vi "4461 timing test.vi"() -> ()   [LabVIEW 2015]
uses:
  <vilib>/DAQmx/write.llb/DAQmx Write (Analog 1D DBL 1Chan NSamp).vi
  <vilib>/DAQmx/create/channels.llb/DAQmx Create Channel (AO-Voltage-Basic).vi
  <vilib>/DAQmx/configure/timing.llb/DAQmx Timing (Sample Clock).vi
  <vilib>/DAQmx/configure/trigger.llb/DAQmx Start Trigger (Digital Edge).vi
  <vilib>/DAQmx/miscellaneous.llb/DAQmx Fill In Error Info.vi
  <resource>/objmgr/daqmx.rc
  <vilib>/Analysis/NI_AALBase.lvlib
panel:
  in  "stop":bool
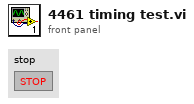
[diagram p1: front panel]
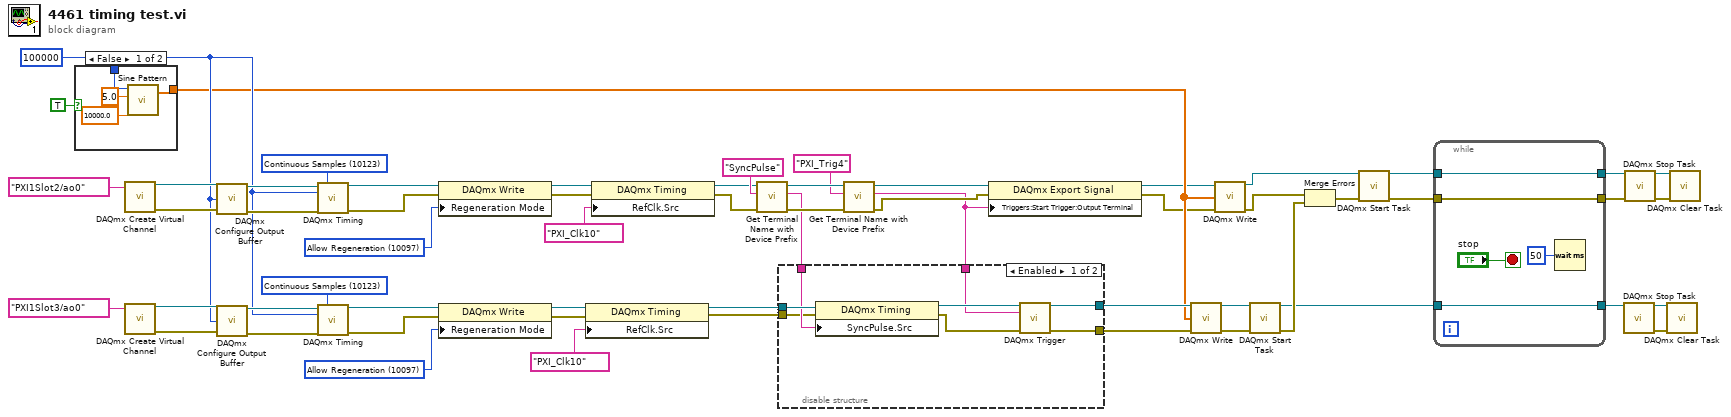
[diagram p0: block diagram]
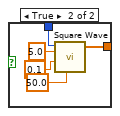
[diagram p2: hidden frame]
diagram:
  w31 = 10123 items=["Finite Samples"=10178, "Continuous Samples"=10123, "Hardware Timed Single Point"=12522] ("sample mode")
  w35 = 10097 items=["Allow Regeneration"=10097, "Do Not Allow Regeneration"=10158] ("RegenMode")
  w30 = 100000
  w51 = 10123 items=["Finite Samples"=10178, "Continuous Samples"=10123, "Hardware Timed Single Point"=12522] ("sample mode")
  w55 = 10097 items=["Allow Regeneration"=10097, "Do Not Allow Regeneration"=10158] ("RegenMode")
  n1 = case shown="False" TRUE {
    tunnel: w30 -> [w62 w68]
    tunnel: [w63 w67] -> w6
    frame False {
      n2 = call <vilib>:"Sine Pattern.vi"("cycles"=10000.0, "amplitude"=5.0, "samples"=w62) -> ("Sinusoidal Pattern"=w63:dbl[])  [unwired: 1 in, 1 out]
    }
    frame True {
      n3 = call <vilib>:"Square Wave.vi"("samples"=w68, "amplitude"=5.0, "frequency"=0.1 ("cycles"), "duty cycle (%)"=50.0) -> ("square wave"=w67:dbl[])  [unwired: 2 in, 2 out]
    }
  }
  n4 = call-poly <vilib>:"DAQmx Create Virtual Channel.vi"("physical channels"=tag "PXI1Slot2/ao0") -> ("task out"=w59:refnum<k21>, "error out"=w54:errorcluster)  [unwired: 13 in]
  n5 = call-poly <vilib>:"DAQmx Create Virtual Channel.vi"("physical channels"=tag "PXI1Slot3/ao0") -> ("task out"=w39:refnum<k21>, "error out"=w34:errorcluster)  [unwired: 13 in]
  n6 = call <vilib>:"DAQmx Configure Output Buffer.vi"("task/channels in"=w59, "buffer size (in samples per channel)"=w30, "error in"=w54) -> ("task out"=w58:refnum<k21>, "error out"=w53:errorcluster)  [unwired: 11 in]
  n7 = call <vilib>:"DAQmx Configure Output Buffer.vi"("task/channels in"=w39, "buffer size (in samples per channel)"=w30, "error in"=w34) -> ("task out"=w38:refnum<k21>, "error out"=w33:errorcluster)  [unwired: 11 in]
  n8 = call-poly <vilib>:"DAQmx Timing.vi"("task/channels in"=w58, "sample mode"=w51, "rate"=w30, "error in"=w53) -> ("task out"=w56:refnum<k21>, "error out"=w57:errorcluster)  [unwired: 10 in]
  n9 = call-poly <vilib>:"DAQmx Timing.vi"("task/channels in"=w38, "sample mode"=w31, "rate"=w30, "error in"=w33) -> ("task out"=w36:refnum<k21>, "error out"=w37:errorcluster)  [unwired: 10 in]
  n10 = property class="DAQmx Write"(reference=w56, error in=w57, "Regeneration Mode"=w55) -> (reference out=w41:refnum<k21>, error out=w40:errorcluster)
  n11 = property class="DAQmx Write"(reference=w36, error in=w37, "Regeneration Mode"=w35) -> (reference out=w28:refnum<k21>, error out=w27:errorcluster)
  n12 = property class="DAQmx Timing"(reference=w28, error in=w27, "RefClk.Src"=tag "PXI_Clk10") -> (reference out=w26:refnum<k21>, error out=w24:errorcluster)
  n13 = property class="DAQmx Timing"(reference=w41, error in=w40, "RefClk.Src"=tag "PXI_Clk10") -> (reference out=w44:refnum<k21>, error out=w43:errorcluster)
  n14 = call "Get Terminal Name with Device Prefix.vi"("error in (no error)"=w43, "Local Terminal Name"="SyncPulse", "task/channels in"=w44) -> ("error out"=w50:errorcluster, "Terminal Name with Device Prefix"=w25:tag, "task out"=w49:refnum<k21>)  [unwired: 6 in]
  n15 = call "Get Terminal Name with Device Prefix.vi"("error in (no error)"=w50, "Local Terminal Name"="PXI_Trig4", "task/channels in"=w49) -> ("error out"=w47:errorcluster, "Terminal Name with Device Prefix"=w11:tag, "task out"=w46:refnum<k21>)  [unwired: 6 in]
  n16 = disable-structure shown="Enabled" {
    disable-tunnel: w26 -> [w76 w78]
    disable-tunnel: w25 -> [w75 _]
    disable-tunnel: w24 -> [w74 w77]
    disable-tunnel: w11 -> [w71 _]
    disable-tunnel: [w70 w77] -> w10
    disable-tunnel: [w69 w78] -> w9
    frame Enabled {
      n17 = property class="DAQmx Timing"(reference=w76, error in=w74, "SyncPulse.Src"=w75) -> (reference out=w73:refnum<k21>, error out=w72:errorcluster)
      n18 = call-poly <vilib>:"DAQmx Trigger.vi"("task/channels in"=w73, "source"=w71, "error in"=w72) -> ("task out"=w69:refnum<k21>, "error out"=w70:errorcluster)  [unwired: 11 in]
    }
    frame Disabled {
    }
  }
  n19 = property class="DAQmx Export Signal"(reference=w46, error in=w47, "Triggers:Start Trigger:Output Terminal"=w11) -> (reference out=w5:refnum<k21>, error out=w3:errorcluster)
  n20 = call-poly <vilib>:"DAQmx Write.vi"("task/channels in"=w9, "data"=w6, "error in"=w10) -> ("task out"=w8:refnum<k21>, "error out"=w7:errorcluster)  [unwired: 10 in, 1 out]
  n21 = call-poly <vilib>:"DAQmx Write.vi"("task/channels in"=w5, "data"=w6, "error in"=w3) -> ("task out"=w4:refnum<k21>, "error out"=w2:errorcluster)  [unwired: 10 in, 1 out]
  n22 = call <vilib>:"DAQmx Start Task.vi"("task/channels in"=w8, "error in"=w7) -> ("task out"=w19:refnum<k21>, "error out"=w23:errorcluster)  [unwired: 12 in]
  n23 = Merge Errors(w2, w23) -> (w22:errorcluster)
  n24 = call <vilib>:"DAQmx Start Task.vi"("task/channels in"=w4, "error in"=w22) -> ("task out"=w20:refnum<k21>, "error out"=w21:errorcluster)  [unwired: 12 in]
  n25 = while {
    tunnel: w21 -> [w80]
    tunnel: w20 -> [w81]
    tunnel: w19 -> [w79]
    tunnel: [w81] -> w18
    tunnel: [w80] -> w17
    tunnel: [w79] -> w16
    stop <- "stop" stop-if-true
    n26 = Wait (ms)(milliseconds to wait=u32 50) -> ()  [unwired: 1 out]
  }
  n27 = call <vilib>:"DAQmx Stop Task.vi"("task/channels in"=w16) -> ("task out"=w13:refnum<k21>, "error out"=w12:errorcluster)  [unwired: 13 in]
  n28 = call <vilib>:"DAQmx Stop Task.vi"("task/channels in"=w18, "error in"=w17) -> ("task out"=w15:refnum<k21>, "error out"=w14:errorcluster)  [unwired: 12 in]
  n29 = call <vilib>:"DAQmx Clear Task.vi"("task in"=w13, "error in"=w12) -> ()  [unwired: 13 in, 1 out]
  n30 = call <vilib>:"DAQmx Clear Task.vi"("task in"=w15, "error in"=w14) -> ()  [unwired: 13 in, 1 out]
